vi "OpenConfig.vi"(8 "error in (no error)":errorcluster, 11 "DAQ_Module in":refnum<class "DAQ_Module.lvclass">) -> (0 "error out":errorcluster, 3 "DAQ_Module out":refnum<class "DAQ_Module.lvclass">)   [LabVIEW 2025, in "DAQ_Module.lvlib" / "DAQ_Module.lvclass"]
uses:
  DAQ_Module.lvclass
  DAQ_Module.lvclass/DAQ_Module.ctl
  Config.vi
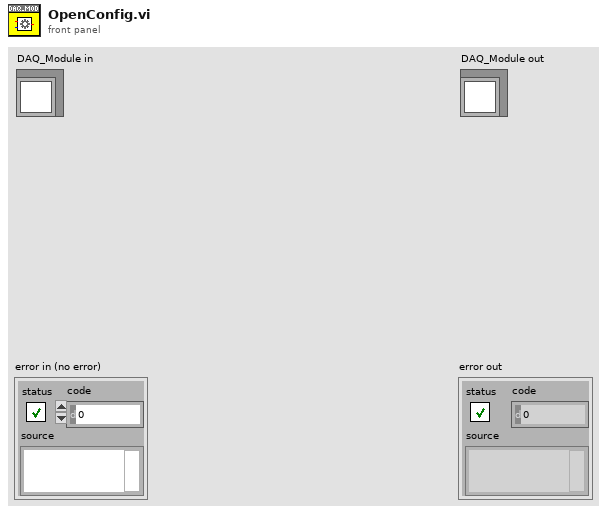
[diagram p1: front panel]
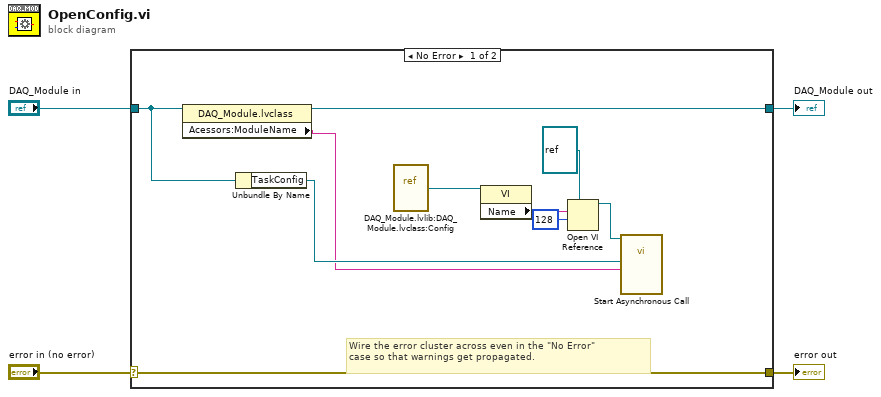
[diagram p0: block diagram]
diagram:
  n1 = case shown="No Error" "error in (no error)" {
    selector: "error in (no error)" -> [w14 w16]
    tunnel: [w14 w16] -> w3
    tunnel: [w13 w15] -> w1
    tunnel: "DAQ_Module in" -> [w12 w15]
    frame No Error {
      # "Wire the error cluster across even in the \"No Error\"\ncase so that warnings get propagated."
      n2 = property class="DAQ_Module.lvclass"(reference=w12) -> (reference out=w13:refnum<class "DAQ_Module.lvclass">, "Acessors:ModuleName"=w5:string)  [unwired: 1 in, 1 out]
      n3 = Unbundle By Name(w12) -> ("TaskConfig"=w6:refnum<data-value>)
      n4 = vi-ref "DAQ_Module.lvlib:DAQ_Module.lvclass:Config.vi"() -> (w11:refnum<vi>)
      n5 = property class="VI"(reference=w11) -> ("Name"=w10:string)  [unwired: 1 in, 2 out]
      n6 = Open VI Reference(type specifier VI Refnum (for type only)=refnum<vi> refnum, vi path=w10, options=128) -> (vi reference=w7:refnum<vi>)  [unwired: 3 in, 1 out]
      n7 = call-by-ref "Start Asynchronous Call"(reference=w7, "Model Name"=w5, "TaskConfig"=w6) -> ()  [unwired: 11 in, 2 out]
    }
    frame Error {
    }
  }
  "error out" <- w3
  "DAQ_Module out" <- w1
